vi "SENS_CORR_EXT_STAT_ON_OFF.vi"(0 "VISA IN":refnum<visa-resource-name>, 1 "Port Ext. ON/OFF":bool, 5 "error in":errorcluster, 7 "Channel":i32) -> (14 "VISA Out":refnum<visa-resource-name>, 19 "error out":errorcluster)   [LabVIEW 2018, in "PNA-X.lvlib"]
doc: "SENSe<cnum>:CORRection:EXTension[:STATe] <ON | OFF> \n(Read-Write) Turns port extensions ON or OFF. \nParameters \n<cnum> Any existing channel number. If unspecified, value is set to 1 \n<ON | OFF> ON (or 1) - turns port extensions ON. \nOFF (or 0) - turns port extensions is OFF. \nExamples SENS:CORR:EXT ON \nsense2:correction:extension:state off \nQuery Syntax SENSe<cnum>:CORRection:EXTension[:STATe]? \nReturn Type Boolean (1 = ON, 0 = OFF) \nDefault OFF \n1708\n\nSense:Correction:Collect:Session Commands \nThe commands in this topic are common to perform both SMC and VMC calibrations. A calibration \nsession is a term used to describe an instance of a SMC or VMC calibration. For more commands, see \nSESS:SMC and SESS:VMC. \nCommands to read (STEP?) and describe (DESC?) each step are provided to facilitate a remote user \ninterface. \nTo perform a NON - SMC or VMC calibration, use either Guided or Mechanical SCPI commands. \nClick on a blue keyword to view the command details. \nSee Also \nSCPI SMC and VMC calibration examples. \nLearn about SMC and VMC calibrations \nSynchronizing the PNA and Controller \nSCPI Command Tree \nSENSe<ch>:CORRection:COLLect:SESSion<n>:ACQuire <step> \n1709\n\n(Write only) Acquire a calibration measurement. \nParameters \n<ch> Any existing channel number. If unspecified, value is set to 1. \n<n> Session number. Choose from 1 to 16. \n<step> Step number to acquire. Use SENS:CORR:COLL:SESS:STEPS? to find the \nnumber of steps required for the calibration. \nExamples SENSe2:CORR:COLL:SESS6:ACQ 5 \nQuery Syntax Not Applicable \nDefault Not Applicable \nSENSe<ch>:CORRection:COLLect:SESSion<n>:CKIT:PORT<p>:CATalog? \n(Read only) Returns a list of cal kits that are compatible with the connector on port <p>. The port \nconnector type is set with SENS:CORR:COLL:SESS:CONN:PORT \nParameters \n<ch> Any existing channel number. If unspecified, value is set to 1. \n<n> Session number. Choose from 1 to 16. \n<p> Port number of connector to query for compatible cal kits. \nExamples SENS2:CORR:COLL:SESS6:CKIT:PORT2:CAT? \nReturn Type Comma separated string values \nDefault Not Applicable \nSENSe<ch>:CORRection:COLLect:SESSion<n>:CKIT:PORT<p>[:SELect] <calkit> \n1710\n\n(Read-Write) Set or return the Cal Kit for the specified port. Use \nSENS:CORR:COLL:SESS:CKIT:PORT:CAT? to list compatible Cal Kits. \nParameters \n<ch> Any existing channel number. If unspecified, value is set to 1 \n<n> Session number. Choose from 1 to 16. \n<p> Port number for which to set cal kit. \n<calkit> Cal Kit Name \nExamples SENS:CORR:COLL:SESS:CKIT:PORT:SEL 85091A \nSENS2:CORR:COLL:SESS6:CKIT:PORT2:SEL? \nQuery Syntax SENS<ch>:CORR:COLL:SESS<n>:CKIT:PORT<p>[:SEL] ? \nReturn Type String \nDefault Not Applicable \nSENSe<ch>:CORRection:COLLect:SESSion<n>:CONN:PORT<p>[:SEL] <conn> \n(Read-Write) Set the connector type and sex for the specified port number. Catalog valid connector \ntypes using SENS:CORR:COLL:GUID:CONN:CAT? \nParameters \n<ch> Any existing channel number. If unspecified, value is set to 1 \n<n> Session number. Choose from 1 to 16. \n<p> Port number for which to select a connector type. \n<conn> Name of the connector type \nExamples SENS2:CORR:COLL:SESS6:CONN:PORT1:SEL \"N Type\" \nQuery Syntax SENS<ch>:CORR:COLL:SESS<n>:CONN:PORT<p>[:SEL] ? \nReturn Type String \nDefault Not Applicable \nSENSe<ch>:CORRection:COLLect:SESSion<n>:DESC? <step> \n1711\n\n(Read-only) Returns the connection prompt for the step. List the number of steps in the calibration \nusing SENS:CORR:COLL:SESS:STEPS?. \nParameters \n<ch> Any existing channel number. If unspecified, value is set to 1 \n<n> Session number. Choose from 1 to 16. \n<step> Step number \nExamples SENS1:CORR:COLL:SESS6:DESC?3 \nReturn Type Numeric \nDefault Not Applicable \nSENSe<ch>:CORRection:COLLect:SESSion<n>:DONE \n(Write only) Ends the calibration sessions. Use SAVE? to calculate error terms and save the CalSet. \nParameters \n<ch> Any existing channel number. If unspecified, value is set to 1 \n<n> Session number. Choose from 1 to 16. \nExamples SENS1:CORR:COLL:SESS6:DONE \nQuery Syntax Not Applicable \nDefault Not Applicable \nSENSe<ch>:CORRection:COLLect:SESSion<n>:INITiate <string> \n1712\n\n(Write only) Initiates an SMC or VMC calibration session. Use the session number for subsequent \nSMC or VMC commands. \nParameters \n<ch> Any existing channel number. If unspecified, value is set to 1 \n<n> Session number. Choose from 1 to 16. If the session number already exists it \nwill be terminated and a new session initiated. \n<string> Name of the calibration. Choose from: \n\"VMC\" or \"VectorMixerCal.VMCType\" \n\"SMC\" or \"ScalarMixerCal.SMCType\" \nExamples SENS1:CORR:COLL:SESS6:INITiate \"VectorMixerCal.VMCType\" \nQuery Syntax Not Applicable \nDefault Not Applicable \nSENSe<ch>:CORRection:COLLect:SESSion<n>:SAVE? \n(Read only) Finish the SMC or VMC calibration, compute error terms, populate and save the CalSet, \nand return the GUID of the Cal Set. \nNote: The destination (Cal Register or User Cal Set) is determined by the setting of the \nSENS:CORR:PREFerence:CSET:SAVE command. \nParameters \n<ch> Any existing channel number. If unspecified, value is set to 1 \n<n> Session number. Choose from 1 to 16. \nExamples SENS1:CORR:COLL:SESS6:SAVE? \nReturn Type String specifying the GUID of the CalSet produced by this session. \nDefault Not Applicable \nSENSe<ch>:CORRection:COLLect:SESSion<n>:STEPs? \n1713\n\n(Read-only) Returns the number of steps required by the Calibration. \nTo ensure this query always completes successfully, first send the write command: \nSENS:CORR:COLL:SESS:STEP, then send the query. \nParameters \n<ch> Any existing channel number. If unspecified, value is set to 1 \n<n> Session number. Choose from 1 to 16. \nExamples SENS1:CORR:COLL:SESS6:STEPs? \nReturn Type Numeric \nDefault Not Applicable \n1714\n\nSense:Correction:Collect:Session:SMC Commands \nPerforms scalar (SMC) calibration on a frequency converting device. \nClick on a blue keyword to view the command details. \nSee Also \nExample Programs \nLearn about FCA Calibrations \nSynchronizing the PNA and Controller \nSCPI Command Tree \nNOTE: To configure a power meter and sensor see SOURce:POWer: commands. \nSENSe<ch>:CORRection:COLLect:SESSion<n >:SMC:ECAL:CHARacteriza <mod> ,<char> \n1715\n\n(Read-Write) Specifies the ECal module and characterization to be used for the SMC calibration. \nParameters \n<ch> Any existing channel number. If unspecified, value is set to 1 \n<n> Session number. Choose from 1 to 16. Learn about Cal sessions. \n<mod> 1 - Electronic Calibration Module \n<char> Specifies which characterization within the ECal module from which to read \nthe confidence data. \n0 Factory characterization (data that was stored in the ECal module by \nAgilent). Default if not specified. \n1 User characterization #1 \n2 User characterization #2 \n3 User characterization #3 \n4 User characterization #4 \n5 User characterization #5 \nExamples SENS:CORR:COLL:SESS:SMC:ECAL:CHAR 1,2 \nQuery Syntax SENS:CORR:COLL:SESS:SMC:ECAL:CHAR? \nReturn Type Numeric \nDefault 1,0 \nSENSe<ch>:CORRection:COLLect:SESSion<n> :SMC:FSIMulator:NETWork<x>:MODE \n<char> \n1716\n\n(Read-Write) Allows you to embed (add) or de-embed (remove) circuit network effects on the input \nand output of your mixer measurement. Learn more. \nParameters \n<ch> Any existing channel number. If unspecified, value is set to 1 \n<n> Session number. Choose from 1 to 16. Learn about Cal sessions. \n<x> Apply network to input or output of mixer. Choose from: \n1 - Input of mixer \n2 - Output of mixer \n<char> Choose from: \nNONE - Do nothing with effects of S2P file. \nEMBed - Add effects of S2P file from the measurement results. \nDEEMbed - Remove effects of S2P file from the measurement results. \nExamples SENS:CORR:COLL:SESS:SMC:FSIM:NETW1:MODE EMB \nQuery Syntax SENS<ch>:CORRection:COLLect:SESSion<n> \n:SMC:FSIMulator:NETWork<x>:MODE? \nReturn Type Character \nDefault NONE \nSENSe<ch>:CORRection:COLLect:SESSion<n> :SMC:FSIMulator:NETWork<x>:FILename \n<string> \n1717\n\n(Read-Write) Specifies the S2P filename to embed or de-embed on the input or output of your mixer \nmeasurement. Learn more. \nParameters \n<ch> Any existing channel number. If unspecified, value is set to 1 \n<n> Session number. Choose from 1 to 16. Learn about Cal sessions. \n<x> Apply network to input or output of mixer. Choose from: \n1 - Input of mixer \n2 - Output of mixer \n<string> Filename of the S2P used for embedding or de-embedding. Use the full path \nname, file name, and .S2P suffix, enclosed in quotes. \nExamples SENS:CORR:COLL:SESS:SMC:FSIM:NETW1:FIL \"C:\\Program \nFiles\\Agilent\\Network Analyzer\\Documents\\WaveguideAdapt.S2P\" \nQuery Syntax SENS<ch>:CORRection:COLLect:SESSion<n> \n:SMC:FSIMulator:NETWork<x>:FILename? \nReturn Type String \nDefault Not Applicable \nSENSe<ch>:CORRection:COLLect:SESSion<n>:SMC:PWRCal:SRCPort <string> Obsolete \n(Read-Write) Specifies which port to calibrate. \nNote: Beginning with Rev 6.0, this command is no longer necessary. Learn more. Because of \nimproved calibration techniques, Both is always selected although a power meter measurement is \nperformed only on port 1. \nParameters \n<ch> Any existing channel number. If unspecified, value is set to 1 \n<n> Session number. Choose from 1 to 16. Learn about Cal sessions. \n<char> '1' Source port 1 (SMC forward direction) \n'2' Source port 2 (SMC reverse direction \n'BOTH' (both forward and reverse directions) \nExamples SENS:CORR:COLL:SESS:SMC:PWRC:SRCP 'both' \nSENSe2:CORRection:COLLection:SESSion6:SMC:PWRCal:SRCPort '2' \nQuery Syntax SENS:CORR:COLL:SESS:SMC:PWRC:SRCP? \n1718\n\nReturn Type String \nDefault 1 \nSENSe<ch>:CORRection:COLLect:SESSion<n>:SMC:TWOPort:ECAL:ORIentation[:STATe] \n<bool> \n(Read-Write) Sets ECAL Auto-Orientation ON or OFF. If setting auto-orientation OFF, you must \nmanually specify the orientation of the ECAL module with \nSENS:CORR:COLL:SESS:SMC:TWOP:ECAL:PORTmap. \nParameters \n<ch> Any existing channel number. If unspecified, value is set to 1 \n<n> Session number. Choose from 1 to 16. Learn about Cal sessions. \n<bool> 0 = Orientation OFF \n1 = Orientation ON \nExamples SENS:CORR:COLL:SESS:SMC:TWOP:ECAL:ORI 1 \nQuery Syntax SENS:CORR:COLL:SESS:SMC:TWOP:ECAL:ORI? \nReturn Type Boolean \nDefault 1 \nSENSe<ch>:CORRection:COLLect:SESSion<n>:SMC:TWOPort:ECAL:PORTmap <mod>, \n<string> \n(Read-Write) Specifies the manual orientation (which ports of the module are connected to which \nports of the PNA) when auto-orientation is OFF. \nParameters \n<ch> Any existing channel number. If unspecified, value is set to 1 \n<n> Session number. Choose from 1 to 16. Learn about Cal sessions. \n<mod> 1 - Electronic Calibration Module \n<string> Format in the following manner: \nAw,Bx,Cy,Dz \nwhere\nA, B, C, and D are literal ports on the ECAL module \n1719\n\nw,x,y, and z are substituted for PNA port numbers to which the ECAL module port \nis connected. \nPorts of the module which are not used are omitted from the string. \nFor example, on a 4-port ECal module with \nport A connected to PNA port 2 \nport B connected to PNA port 3 \nport C not connected \nport D connected to PNA port 1 \nthe string would be: A2,B3,D1 \nIf either the receive port or source port (or load port for 2-port cal) of the \nCALC:PAR:SELected measurement is not in this string and orientation is OFF, \nan attempt to perform an ECal calibration will fail. \nExamples SENS:CORR:COLL:SESS:SMC:TWOP:ECAL:PORTmap 1,'A1,B2' \nQuery Syntax SENS:CORR:COLL:SESS:SMC:TWOP:ECAL:PORTmap? \nReturn Type String \nDefault \"A1,B2\" \nSENSe<ch>:CORRection:COLLect:SESSion<n >:SMC:TWOPort:METHod <string> \n1720\n\n(Read-Write) Specifies the guided ECal method for performing the thru portion of the calibration. \nParameters \n<ch> Any existing channel number. If unspecified, value is set to 1 \n<n> Session number. Choose from 1 to 16. Learn about Cal sessions. \n<string> ECAL Method: Choose from: \n'DEFAULT' - Default \n'ADAP' - Adapter removal \n'FLUSH' - Flush Through \n'UNKN' - Unknown Thru \nExamples SENS:CORR:COLL:SESS:SMC:TWOPort:METH 'default' \nQuery Syntax SENS:CORR:COLL:SESS:SMC:TWOPort:METH? \nReturn Type String \nDefault DEFAULT \nSENSe<ch>:CORRection:COLLect:SESSion<n >:SMC:TWOPort:OMITisolat <bool> \n(Read-Write) Select to omit or perform the isolation portion of the ECAL. \nParameters \n<ch> Any existing channel number. If unspecified, value is set to 1 \n<n> Session number. Choose from 1 to 16. Learn about Cal sessions. \n<bool> 1 - Omit isolation \n0 - Perform isolation \nExamples SENS:CORR:COLL:SESS:SMC:TWOPort:OMIT 1 \nQuery Syntax SENS:CORR:COLL:SMC:TWOPort:OMIT? \nReturn Type Boolean \nDefault 1 \nSENSe<ch>:CORRection:COLLect:SESSion<n >:SMC:TWOPort:OPTion <string> \n1721\n\n(Read-Write) Sets the SMC calibration to ECAL or MECHanical \nParameters \n<ch> Any existing channel number. If unspecified, value is set to 1 \n<n> Session number. Choose from 1 to 16. Learn about Cal sessions. \n<char> Choose from: \n'ECAL' Electronic Calibration Module \n'MECH' Mechanical Calibration Kit \nExamples SENS:CORR:COLL:SESS:SMC:TWOPort:OPTion 'ECAL' \nQuery Syntax SENS:CORR:COLL:SESS:SMC:TWOPort:OPTion? \nReturn Type String \nDefault ECAL \n1722\n\nSense:Correction:Collect:Session:VMC Commands \nPerforms a vector (VMC) calibration on a frequency converting device. \nClick on a blue keyword to view the command details. \nSee Also \nExample Programs \nLearn about VMC Calibration \nSynchronizing the PNA and Controller \nSENSe<ch>:CORRection:COLLect:SESSion<n> :VMC:FSIMulator:NETWork<x>:MODE \n<char> \n1723\n\n(Read-Write) Allows you to embed (add) or de-embed (remove) circuit network effects on the input \nand output of your mixer measurement. Learn more. \nParameters \n<ch> Any existing channel number. If unspecified, value is set to 1 \n<n> Session number. Choose from 1 to 16. Learn about Cal sessions. \n<x> Apply network to input or output of mixer. Choose from: \n1 - Input of mixer \n2 - Output of mixer \n<char> Choose from: \nNONE - Do nothing with effects of S2P file. \nEMBed - Add effects of S2P file from the measurement results. \nDEEMbed - Remove effects of S2P file from the measurement results. \nExamples SENS:CORR:COLL:SESS:VMC:FSIM:NETW1:MODE EMB \nQuery Syntax SENS<ch>:CORRection:COLLect:SESSion<n> \n:VMC:FSIMulator:NETWork<x>:MODE? \nReturn Type Character \nDefault NONE \nSENSe<ch>:CORRection:COLLect:SESSion<n> :VMC:FSIMulator:NETWork<x>:FILename \n<string> \n1724\n\n(Read-Write) Specifies the S2P filename to embed or de-embed on the input or output of your mixer \nmeasurement. Learn more. \nParameters \n<ch> Any existing channel number. If unspecified, value is set to 1 \n<n> Session number. Choose from 1 to 16. Learn about Cal sessions. \n<x> Apply network to input or output of mixer. Choose from: \n1 - Input of mixer \n2 - Output of mixer \n<string> Filename of the S2P used for embedding or de-embedding. Use the full path \nname, file name, and .S2P suffix, enclosed in quotes. \nExamples SENS:CORR:COLL:SESS:VMC:FSIM:NETW1:FIL \"C:\\Program \nFiles\\Agilent\\Network Analyzer\\Documents\\WaveguideAdapt.S2P\" \nQuery Syntax SENS<ch>:CORRection:COLLect:SESSion<n> \n:VMC:FSIMulator:NETWork<x>:FILename? \nReturn Type String \nDefault Not Applicable \nSENSe<ch>:CORRection:COLLect:SESSion<n> :VMC:MIXer:CHARacterize:CAL:FILename \n<string> \n(Read-Write) Specifies the .S2P filename used for mixer characterization. Use the \nVMC:MIXer:CHARacterize:CAL: OPTion command to recall the file for mixer characterization. \nOnce recalled, use this command to query the current filename or set a new filename. \nParameters \n<ch> Any existing channel number. If unspecified, value is set to 1 \n<n> Session number. Choose from 1 to 16. Learn about Cal sessions. \n<string> Filename of the S2P used for mixer characterization. Use the full path name, \nfile name, and .S2P suffix, enclosed in quotes. \nExamples SENS2:CORR:COLL:SESS4:VMC:MIXer:CHAR:CAL:FILE \"C:\\Program \nFiles\\Agilent\\Network Analyzer\\Documents\\MyMixer.S2P\" \nQuery Syntax SENS:CORR:COLL:SESS:VMC:MIX:CHAR:CAL:FIL? \nReturn Type String \nDefault C:\\Program Files\\Agilent\\Network Analyzer\\Documents\\default.s2p \n1725\n\nSENSe<ch>:CORRection:COLLect:SESSion<n> :VMC:MIXer:CHARacterize:CAL: OPTion \n<char> \n(Read-Write) Sets the mixer characterization method to ECal, Mechanical, or read from a file. \nParameters \n<ch> Any existing channel number. If unspecified, value is set to 1 \n<n> Session number. Choose from 1 to 16. Learn about Cal sessions. \n<char> ECAL - Electronic Calibration Module \nMECH - Mechanical Calibration Kit \nFILE, <filename> - Retrieve a mixer characterization file. Also specify the \nfilename of the S2P used for mixer characterization. Use the full path name, \nfile name, and .S2P suffix. Use the VMC:CHARacterize:CAL:FILename \ncommand to query the filename.. \nExamples SENS:CORR:COLL:SESS:VMC:MIX:CHAR:CAL:OPT ECAL \nSENS2:CORR:COLL:SESS6:VMC:MIXer:CHAR:CAL:OPTion FILE, \nMyMixerFile.mxr \nQuery Syntax SENS:CORR:COLL:SESS:VMC:MIX:CHAR:CAL:OPT? \nReturn Type String \nDefault MECH \nSENSe<ch>:CORRection:COLLect:SESSion<n> :VMC:MIXer:CHARacterize:CAL: REVerse \n<bool> \n(Read-Write) Specifies the direction in which to characterize the calibration mixer. Learn more about \nthe calibration mixer. \nParameters \n<ch> Any existing channel number. If unspecified, value is set to 1 \n<n> Session number. Choose from 1 to 16. Learn about Cal sessions. \n<bool> False (0) - Characterize the calibration mixer in the SAME direction as that \nspecified in the mixer setup. \nTrue (1) - Characterize the calibration mixer in the REVERSE direction as that \nspecified in the mixer setup. \nExamples SENS:CORR:COLL:SESS:VMC:MIX:CHAR:CAL:REV 1 \n1726\n\nQuery Syntax SENS:CORR:COLL:SESS:VMC:MIX:CHAR:CAL:REV? \nReturn Type Boolean \nDefault False \nSENSe<ch>:CORRection:COLLect:SESSion<n > :VMC:MIXer:ECAL:CHARacteriza <mod> \n,<char> \n(Read-Write) Specifies the ECal module and characterization to be used for the mixer characterization \nportion of the calibration. \nParameters \n<ch> Any existing channel number. If unspecified, value is set to 1 \n<n> Session number. Choose from 1 to 16. Learn about Cal sessions. \n<mod> 1 - Electronic Calibration Module \n<char> Characterization number in the specified ECAL module. Choose from: \n0 Factory characterization (data that was stored in the ECal module by \nAgilent). Default if not specified. \n1 User characterization #1 \n2 User characterization #2 \n3 User characterization #3 \n4 User characterization #4 \n5 User characterization #5 \nExamples SENS:CORR:COLL:SESS:VMC:MIX:ECAL:CHAR 1,0 \nQuery Syntax SENS:CORR:COLL:SESS:VMC:MIX:ECAL:CHAR? \nReturn Type Numeric \nDefault 1,0 \nSENSe<ch>:CORRection:COLLect:SESSion<n> :VMC:MIXer:ECAL:PORTmap <mod>, \n<string> \n1727\n\n(Read-Write) Sets the port mapping for the mixer characterization with ECal. This command is \nrequired if SENS:CORR:COLL:SESS:VMC:MIX:CHAR:CAL:OPT ECAL is specified. \nParameters \n<ch> Any existing channel number. If unspecified, value is set to 1 \n<n> Session number. Choose from 1 to 16. Learn about Cal sessions. \n<mod> 1 - Electronic Calibration Module \n<string> Choose from: \n\"A1\" - ECAL module port A is connected to PNA port 1 \n\"B1\" - ECAL module port B is connected to PNA port 1 \nExamples SENS:CORR:COLL:SESS:VMC:MIX:ECAL:PORT? \nSENS2:CORR:COLL:SESS:VMC:MIXer:ECAL:PORTmap 1,\"A1\" \nQuery Syntax SENS:CORR:COLL:SESS:VMC:MIX:ECAL:PORTmap? \nReturn Type String \nDefault \"A1\" \nSENSe<ch>:CORRection:COLLect:SESSion<n>:VMC:OPERation <string> \n(Read-Write) Perform either full VMC calibration or mixer characterization only. \nParameters \n<ch> Any existing channel number. If unspecified, value is set to 1 \n<n> Session number. Choose from 1 to 16. Learn about Cal sessions. \n<char> 'CAL' - full calibration and mixer characterization \n'CHAR' - mixer characterization only (no reference mixer required) - Saves \nan .S2P file with the filename specified in \nSENS<ch>:CORR:COLL:SESSion<n >:VMC:CHARacterize:CAL:FILename \n<filename> . If none is specified, a filename is automatically generated and can \nbe queried using the filename command. \nExamples SENS:CORR:COLL:SESS:VMC:OPER 'CAL' \nQuery Syntax SENS:CORR:COLL:SESS:VMC:OPER? \nReturn Type String \nDefault CAL \n1728\n\nSENSe<ch>:CORRection:COLLect:SESSion<n> :VMC:TWOPort:ECAL:CHARacteriza <mod> \n,<char> \n(Read-Write) Specifies the ECal module and characterization to be used for the VMC calibration. \nParameters \n<ch> Any existing channel number. If unspecified, value is set to 1 \n<n> Session number. Choose from 1 to 16. Learn about Cal sessions. \n<mod> 1 - Electronic Calibration Module \n<char> Characterization number in the specified ECAL module. Choose from: \n0 Factory characterization (data that was stored in the ECal module by \nAgilent). Default if not specified. \n1 User characterization #1 \n2 User characterization #2 \n3 User characterization #3 \n4 User characterization #4 \n5 User characterization #5 \nExamples SENS:CORR:COLL:SESS:VMC:TWOP:ECAL:CHAR 1,1 \nQuery Syntax SENS:CORR:COLL:SESS:VMC:TWOP:ECAL:CHAR? \nReturn Type Integer \nDefault 1,0 \nSENSe<ch>:CORRection:COLLect:SESSion<n> :VMC:TWOPort:ECAL:ORIentation[:STATe] \n<bool> \n1729\n\n(Read-Write) Sets ECAL orientation for the VMC ECal. \nParameters \n<ch> Any existing channel number. If unspecified, value is set to 1 \n<n> Session number. Choose from 1 to 16. Learn about Cal sessions. \n<bool> 1 = ON \n0 = OFF \nExamples SENS:CORR:COLL:SESS:VMC:TWOP:ECAL:ORI 1 \nQuery Syntax SENS:CORR:COLL:SESSion:VMC:TWOPort:ECAL:ORIentation[:STATe]? \nReturn Type Integer \nDefault ON \nSENSe<ch>:CORRection:COLLect:SESSion<n> :VMC:TWOPort:ECAL:PORTmap <mod>, \n<string> \n(Read-Write) Specifies the manual orientation (which ports of the module are connected to which \nports of the PNA) when orientation is turned off. \nParameters \n<ch> Any existing channel number. If unspecified, value is set to 1 \n<n> Session number. Choose from 1 to 16. Learn about Cal sessions. \n<mod> 1 - Electronic Calibration Module \n<string> Port Map, formatted in the following manner: \nAw,Bx,Cy,Dz \nwhere: \nA, B, C, and D are literal ports on the ECAL module. \nw,x,y, z are substituted for PNA port numbers to which the ECAL module port is \nconnected. \nPorts of the module which are not used are omitted from the string. \nFor example, on a 4-port ECal module with: \nport A connected to PNA port 2 \n1730\n\nport B connected to PNA port 3 \nport C not connected \nport D connected to PNA port 1 \nthe string would be: A2,B3,D1 \nIf either the receive port or source port (or load port for 2-port cal) of the \nmeasurement is not in this string and orientation is OFF, an attempt to perform \nan ECal will fail. \nExamples SENS:CORR:COLL:SESS:VMC:TWOP:ECAL:PORTmap 1,\"A2,B1\" \nQuery Syntax SENS:CORR:COLL:SESS:VMC:TWOP:ECAL:PORTmap? \nReturn Type string \nDefault \"A1,B2\" \nSENSe<ch>:CORRection:COLLect:SESSion<n> :VMC:TWOPort:METHod <string> \n(Read-Write) Specifies the guided ECal method for performing the thru portion of the calibration. \nParameters \n<ch> Any existing channel number. If unspecified, value is set to 1 \n<n> Session number. Choose from 1 to 16. Learn about Cal sessions. \n<char> 'DEFAULT' - Default \n'ADAP' - Adapter removal \n'FLUSH' - Flush Through \n'UNKN' - Unknown Thru \nExamples SENS:CORR:COLL:SESS:VMC:TWOP:METH 'ADAP' \nSENSe2:CORR:COLL:SESSion6:VMC:TWOPort:METHod 'FLUSH' \nQuery Syntax SENS:CORR:COLL:SESS:VMC:TWOP:METH? \nReturn Type String \nDefault DEFAULT \nSENSe<ch>:CORRection:COLLect:SESSion<n> :VMC:TWOPort:OMITisolat <bool> \n1731\n\n(Read-Write) Select to omit or perform the isolation portion of the ECAL. \nParameters \n<ch> Any existing channel number. If unspecified, value is set to 1 \n<n> Session number. Choose from 1 to 16. Learn about Cal sessions. \n<bool> 1 - omit isolation \n0 - perform isolation \nExamples SENS:CORR:COLL:SESS:VMC:TWOP:OMIT 1 \nQuery Syntax SENS:CORR:COLL:SESS:VMC:TWOP:OMIT? \nReturn Type Numeric \nDefault 1 \nSENSe<ch>:CORRection:COLLect:SESSion<n> :VMC:TWOPort:OPTion <string> \n(Read-Write) Sets the 2-port calibration option to ECAL or MECHanical \nParameters \n<ch> Any existing channel number. If unspecified, value is set to 1 \n<n> Session number. Choose from 1 to 16. Learn about Cal sessions. \n<char> \nChoose from: \n'ECAL' Electronic Calibration Module \n'MECH' Mechanical Calibration Kit \nExamples SENS:CORR:COLL:SESS:VMC:TWOP:OPT 'MECH' \nSENSe2:CORR:COLL:SESSion6:VMC:TWOPort:OPTion 'ECAL' \nQuery Syntax SENS:CORR:COLL:SESS:VMC:TWOP:OPT? \nReturn Type String \nDefault \"MECH\" \n1732\n\nSense:Couple Commands \nClick on a blue keyword to view the command details. \nSee Also \nExample Programs \nSynchronizing the PNA and Controller \nSCPI Command Tree"
uses:
  PNA-X.lvlib
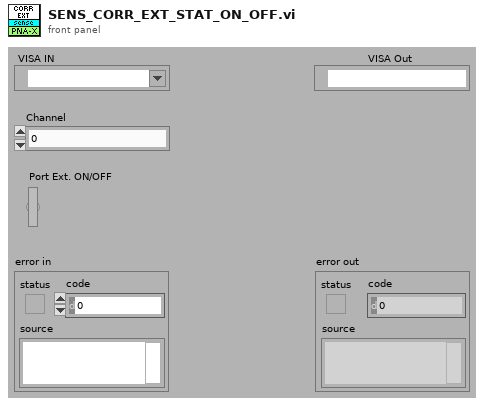
[diagram p1: front panel]
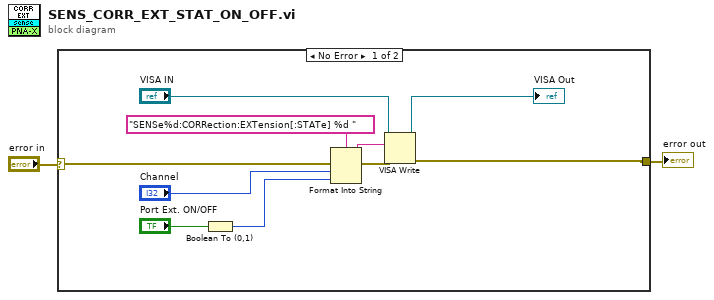
[diagram p0: block diagram]
diagram:
  n1 = case shown="No Error" "error in" {
    selector: "error in" -> [w12 w13]
    tunnel: [w7 w13] -> w1
    frame No Error {
      n2 = Boolean To (0,1)(Boolean="Port Ext. ON/OFF") -> (0, 1=w3:i16)
      n3 = Format Into String(format string="SENSe%d:CORRection:EXTension[:STATe] %d " ("Cmdline"), error in=w12, "Channel", w3) -> (resulting string=w10:string, error out=w11:errorcluster)  [unwired: 1 in]
      n4 = VISA Write(VISA resource name="VISA IN", write buffer=w10, error in (no error)=w11) -> (VISA resource name out=→"VISA Out":refnum<visa-resource-name>, error out=w7:errorcluster)  [unwired: 1 out]
    }
    frame Error {
    }
  }
  "error out" <- w1
